vi "Read Data.vi"(5 "CS (None)":refnum<class "SPI CS.lvclass">, 7 "SPI":refnum<class "SPI.lvclass">, 8 "error in (no error)":errorcluster, 9 "Len":u8, 11 "Session In":refnum<class "Session.lvclass">) -> (0 "error out":errorcluster, 1 "Data":string, 3 "Session Out":refnum<class "Session.lvclass">)   [LabVIEW 2024, in "CTI.lvlib" / "SPI.lvclass"]
uses:
  SPI.lvclass
  Session/Session.lvclass
  SPI CS/SPI CS.lvclass
  SPI.lvclass/SPI.ctl
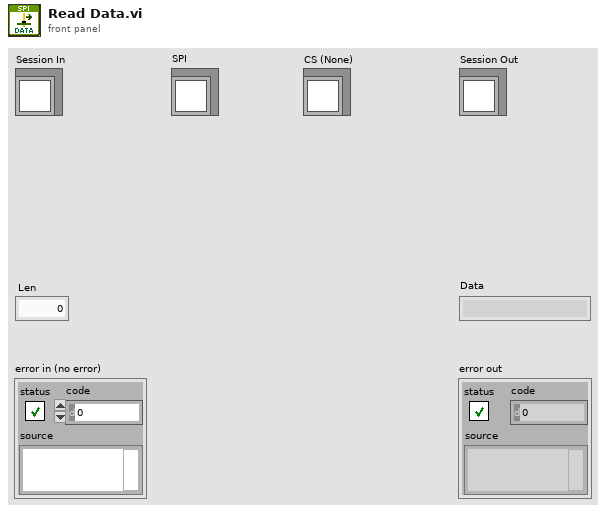
[diagram p1: front panel]
types:
  T1 = typedef "CTI.lvlib/SPI Number.ctl" = i8
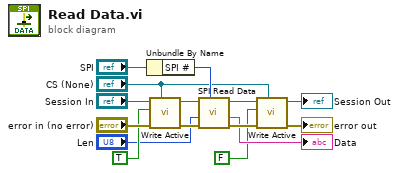
[diagram p0: block diagram]
diagram:
  n1 = Unbundle By Name("SPI") -> ("SPI #"=w7:T1)
  n2 = call "Write Active.vi"("SPI CS"="CS (None)", "error in (no error)"="error in (no error)", "Active"=TRUE, "Session In"="Session In") -> ("error out"=w11:errorcluster, "Session Out"=w10:refnum<class "Session.lvclass">)  [unwired: 6 in]
  n3 = call "SPI Read Data.vi"("SPI #"=w7, "error in (no error)"=w11, "Len"="Len", "Session in"=w10) -> ("error out"=w15:errorcluster, "Data"=→"Data":string, "Session out"=w5:refnum<class "Session.lvclass">)  [unwired: 5 in]
  n4 = call "Write Active.vi"("SPI CS"="CS (None)", "error in (no error)"=w15, "Active"=FALSE, "Session In"=w5) -> ("error out"=→"error out":errorcluster, "Session Out"=→"Session Out":refnum<class "Session.lvclass">)  [unwired: 6 in]
